vi "Move Item in Tree.vi"(7 "Tree ref":refnum<vi>, 8 "Insertion indent":i32, 9 "Tree Move Indices":T1[](array[typedef]), 10 "Insertion index":i32, 11 "TreeItems (current)":T2[](array[typedef])) -> (0 "error out":errorcluster)   [LabVIEW 2020, in "BetterDragAndDrop.lvlib" / "BetterTreeHandle.lvclass"]
uses:
  BetterTreeHandle/BetterTreeHandle.lvclass
  TreeItem.ctl
  Tree Move Indices.ctl
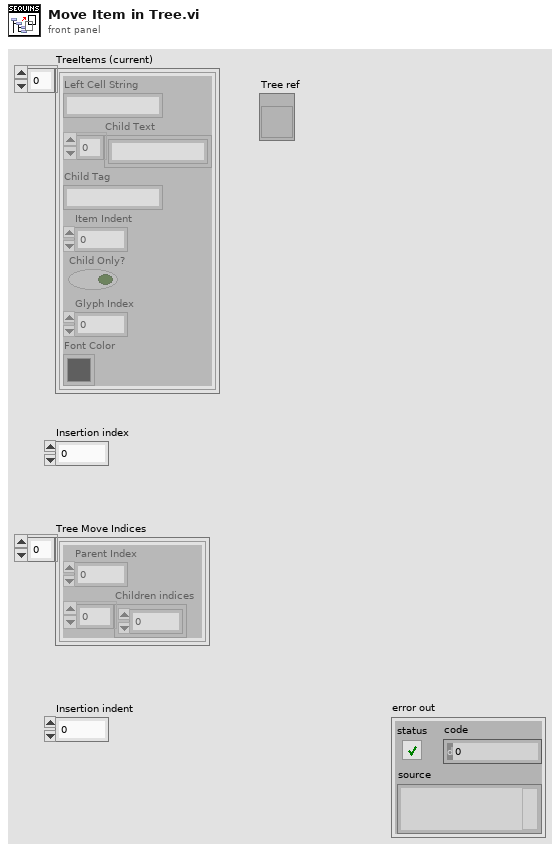
[diagram p1: front panel]
types:
  T1 = typedef "BetterDragAndDrop.lvlib/BetterTreeHandle.lvclass/Tree Move Indices.ctl" = cluster{"Parent Index":i32, "Children indices":i32[]}
  T2 = typedef "BetterDragAndDrop.lvlib/BetterTreeHandle.lvclass/TreeItem.ctl" = cluster{"Left Cell String":string, "Child Text":string[], "Child Tag":string, "Item Indent":i32, "Child Only?":bool, "Glyph Index":i32, "Font Color":u32}
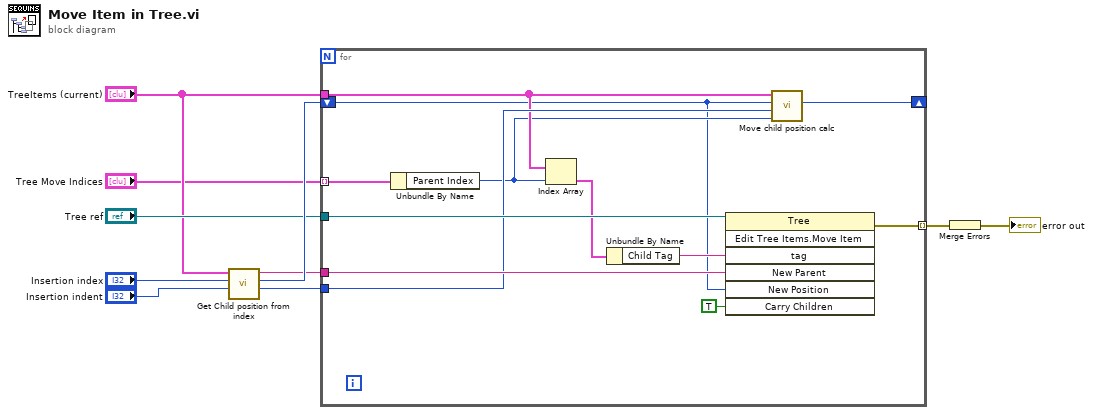
[diagram p0: block diagram]
diagram:
  n1 = call "Get Child position from index.vi"("Insertion indent"="Insertion indent", "Insertion index"="Insertion index", "TreeItems (current)"="TreeItems (current)") -> ("Parent Tag Index"=w8:i32, "Child Position"=w10:i32, "Parent Tag"=w7:string)  [unwired: 6 in]
  n2 = for {
    tunnel: "Tree ref" -> [w22]
    tunnel: w7 -> [w21]
    tunnel: "Tree Move Indices" -> [w20] mode=indexing
    tunnel: "TreeItems (current)" -> [w14]
    shift-right: [w16] -> _
    shift-left: w10 -> [w12]
    tunnel: w8 -> [w15]
    tunnel: [w11] -> w6 mode=indexing
    n3 = Unbundle By Name(w20) -> ("Parent Index"=w13:i32)
    n4 = Index Array(array=w14, index=w13) -> (element=w19:T2)
    n5 = Unbundle By Name(w19) -> ("Child Tag"=w18:string)
    n6 = invoke class="Tree" method="Edit Tree Items.Move Item"(reference=w22, "tag"=w18, "New Parent"=w21, "New Position"=w12, "Carry Children"=TRUE ("Carry Children?")) -> (error out=w11:errorcluster)  [unwired: 2 in, 6 out]
    n7 = call "Move child position calc.vi"("Index to move"=w13, "Insertion Parent Tag Index"=w15, "Insertion Position"=w12, "TreeItems"=w14) -> ("Insertion Position (next loop)"=w16:i32)  [unwired: 7 in]
  }
  n8 = Merge Errors(w6) -> (→"error out":errorcluster)
